vi "总磷氨氮测量流程.vi"(10 "量程模式":T1, 11 "参数":T2={"站号"=1, "量程切换"=enum."AUTO", "控制命令"=enum."启动测量", "模式设置"=enum."待机", "测量间隔"=0} {"站号" items=["总磷"=1, "总氮"=2]}) -> ()   [LabVIEW 2016, in "斯坦道仪器.lvlib"]
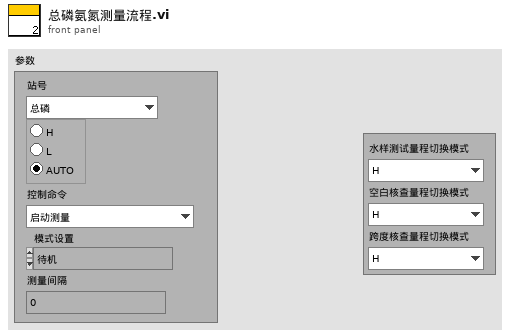
[diagram p1: front panel]
types:
  T1 = cluster{"水样测试量程切换模式":enum16{"H", "L", "AUTO"}, "空白核查量程切换模式":enum16{"H", "L", "AUTO"}, "跨度核查量程切换模式":enum16{"H", "L", "AUTO"}}
  T2 = cluster{"站号":u16, "量程切换":enum32{"H", "L", "AUTO"}, "控制命令":enum16{"启动测量", "标样核查", "零点核查", "跨度核查", "空白测试", "平行样测试", "加标回收", "空白校准", "标样校准", "初始化（清洗）", "停止测试", "仪器重启", "校时", "模式设置", "测量间隔设置"}, "模式设置":enum16{"待机", "连续模式", "周期模式", "定点模式", "受控模式", "手动模式"}, "测量间隔":u16}
  T3 = enum16{"初始化", "通电", "参数1启动", "等待参数1测试完成", "参数1测试完成", "参数1存储数据", "参数2启动", "等待参数2测试完成", "参数2测试完成", "参数2存储数据", "断电", "结束"}
  T4 = cluster{"时间标识":timestamp, "设备":string, "日志信息":string, "流程参数":string}
  T5 = cluster{"时间标识":timestamp, "监测值":sgl, "单位":u16, "数据标识":string, "因子编码":u32, "标样参考值":sgl, "F0":sgl, "F1":sgl, "F2":sgl, "F3":sgl, "F4":sgl, "F5":sgl, "F6":sgl, "F7":sgl, "X":sgl, "温度":sgl, "湿度":sgl, "量程标识":string}
  T6 = enum16{"维护数据", "水样测试", "标样核查", "零点核查", "跨度核查", "空白测试", "平行样测试", "加标回收", "空白校准", "标样校准", "初始化（清洗）"}
  T7 = cluster{"系统时间":timestamp, "工作状态":enum16{"空闲", "水样测试", "标样核查", "零点核查", "跨度核查", "空白测试", "平行样测试", "加标回收", "空白校准", "标样校准", "初始化（清洗）"}, "测量模式":enum16{"待机", "连续模式", "周期模式", "定点模式", "受控模式", "手动模式"}, "告警代码":enum16{"无告警", "缺试剂告警", "缺水样告警", "缺蒸馏水告警", "缺标液告警", "仪表漏液告警", "标定异常告警", "超量程告警", "加热异常", "低试剂预警", "超上限告警", "超下限告警", "仪表内部其他异常", "滴定异常告警", "电极异常告警", "量程切换告警", "参数设置告警", "PH电极电位异常", "电导率电极异常", "浊度光度异常", "溶解氧电极异常", "溶解氧光强异常", "温度异常告警", "PH异常告警", "溶解氧异常告警", "电导率异常告警", "浊度异常告警", "叶绿素异常告警", "藻密度异常告警", "蓝绿藻异常告警", "ORP异常告警", "氨氮异常告警", "清洁刷异常告警", "SD卡异常告警", "蓝牙异常告警", "Wifi异常告警", "流程异常告警"}, "故障代码":enum16{"无故障", "电机故障", "温度故障", "通讯故障", "滴定故障"}, "日志代码":u16, "软件版本":u16, "F0":sgl, "F1":sgl, "F2":sgl, "F3":sgl, "T":sgl, "H":sgl, "id":u16, "flowid":u16, "量程":u16, "总磷控温温度1":sgl, "营养盐控温温度2":sgl, "ADC":sgl}
  T8 = enum16{"启动测量", "标样核查", "零点核查", "跨度核查", "空白测试", "平行样测试", "加标回收", "空白校准", "标样校准", "初始化（清洗）", "停止测试", "仪器重启", "校时", "模式设置", "测量间隔设置"}
  T9 = enum16{"空闲", "水样测试", "标样核查", "零点核查", "跨度核查", "空白测试", "平行样测试", "加标回收", "空白校准", "标样校准", "初始化（清洗）"}
  T10 = cluster{"因子编码":u32, "单位":u16, "标样参考值":sgl, "水样数据时间":timestamp, "水样实测值":sgl, "水样数据标识":string, "标样数据时间":timestamp, "标样实测值":sgl, "标样数据标识":string, "空白数据时间":timestamp, "空白实测值":sgl, "空白数据标识":string, "零点核查数据时间":timestamp, "零点核查实测值":sgl, "零点核查数据标识":string, "跨度核查数据时间":timestamp, "跨度核查实测值":sgl, "跨度核查数据标识":string, "加标回收数据时间":timestamp, "加标回收实测值":sgl, "加标回收数据标识":string, "平行样数据时间":timestamp, "平行样实测值":sgl, "平行样数据标识":string, "F0":sgl, "F1":sgl, "F2":sgl, "F3":sgl, "F4":sgl, "F5":sgl, "F6":sgl, "F7":sgl, "温度":sgl, "湿度":sgl, "X值":sgl}
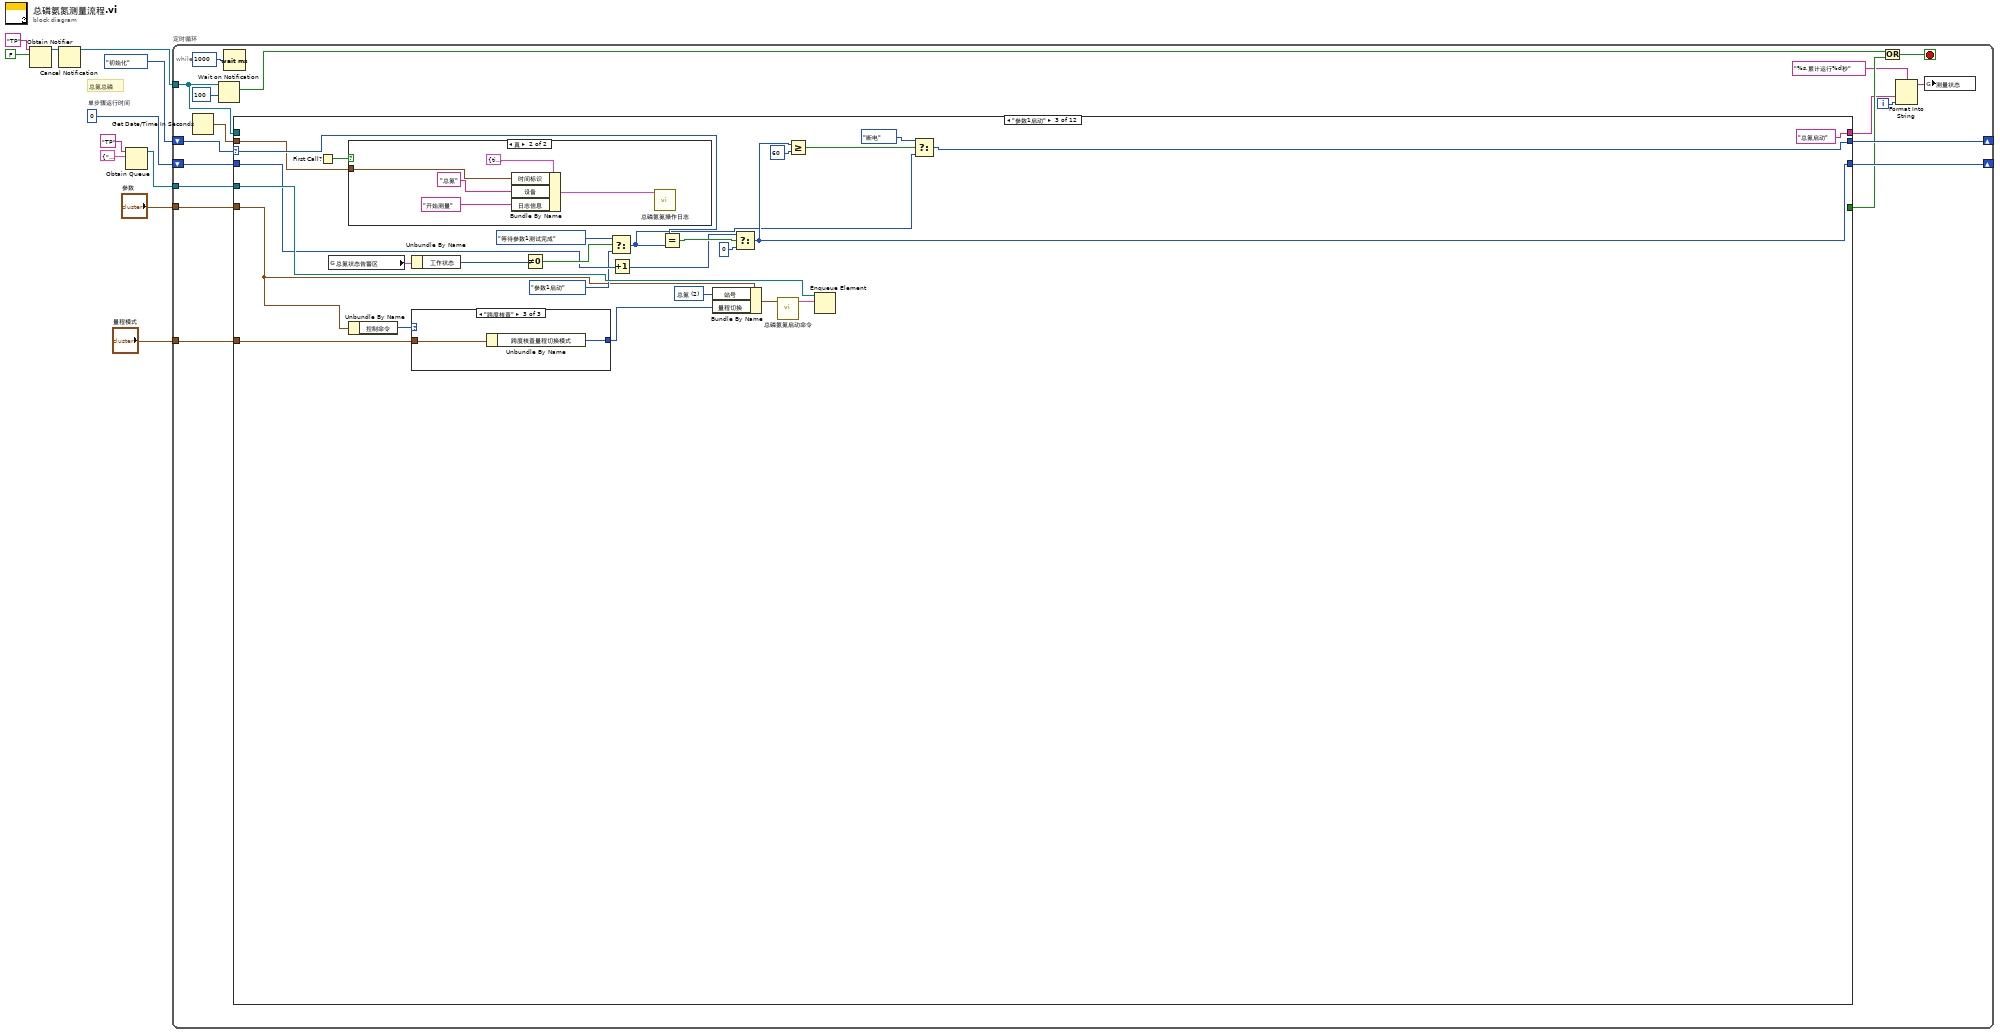
[diagram p0: block diagram]
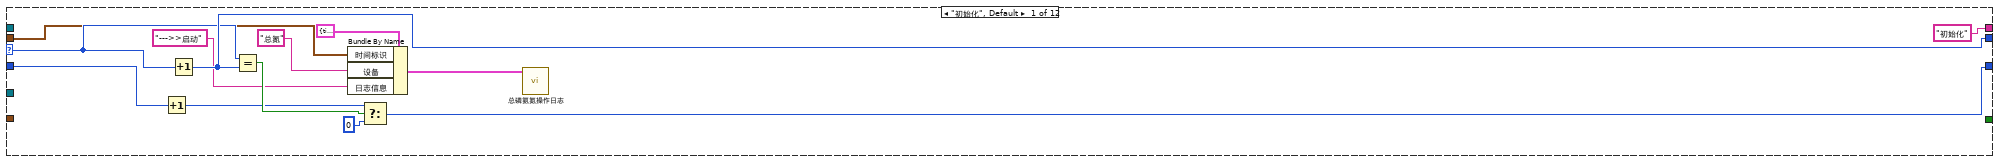
[diagram p2: hidden frame]
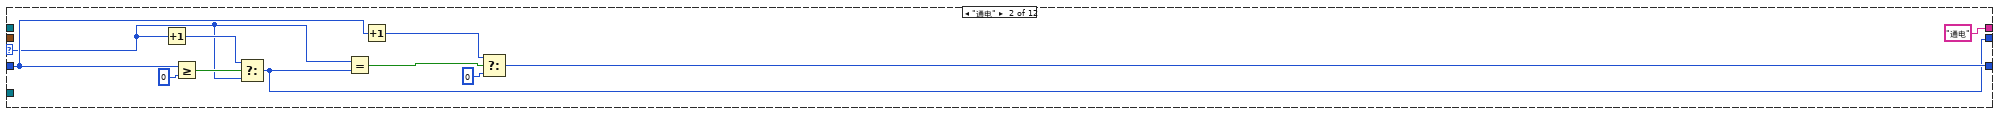
[diagram p3: hidden frame]
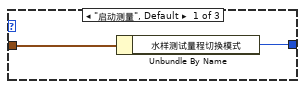
[diagram p4: hidden frame]
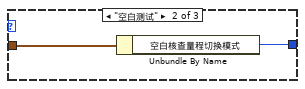
[diagram p5: hidden frame]
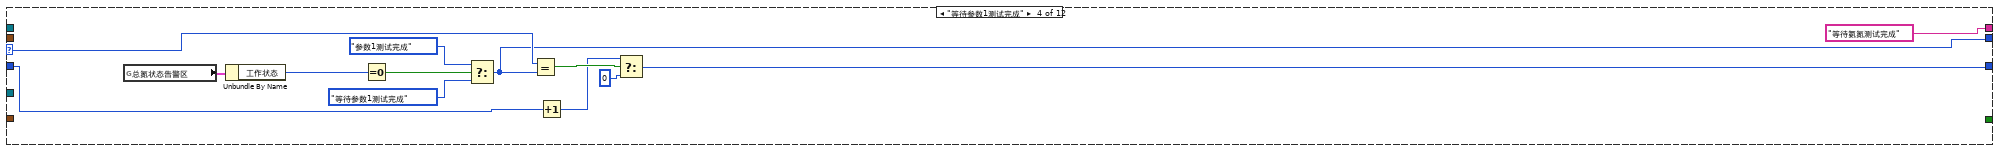
[diagram p7: hidden frame]
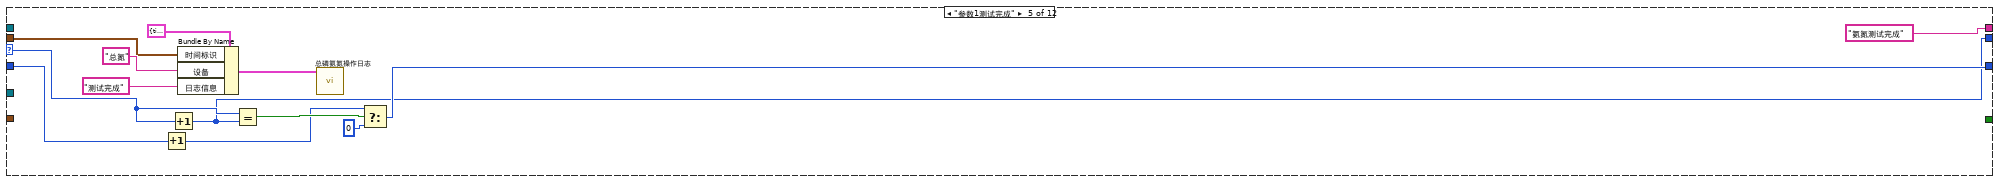
[diagram p8: hidden frame]
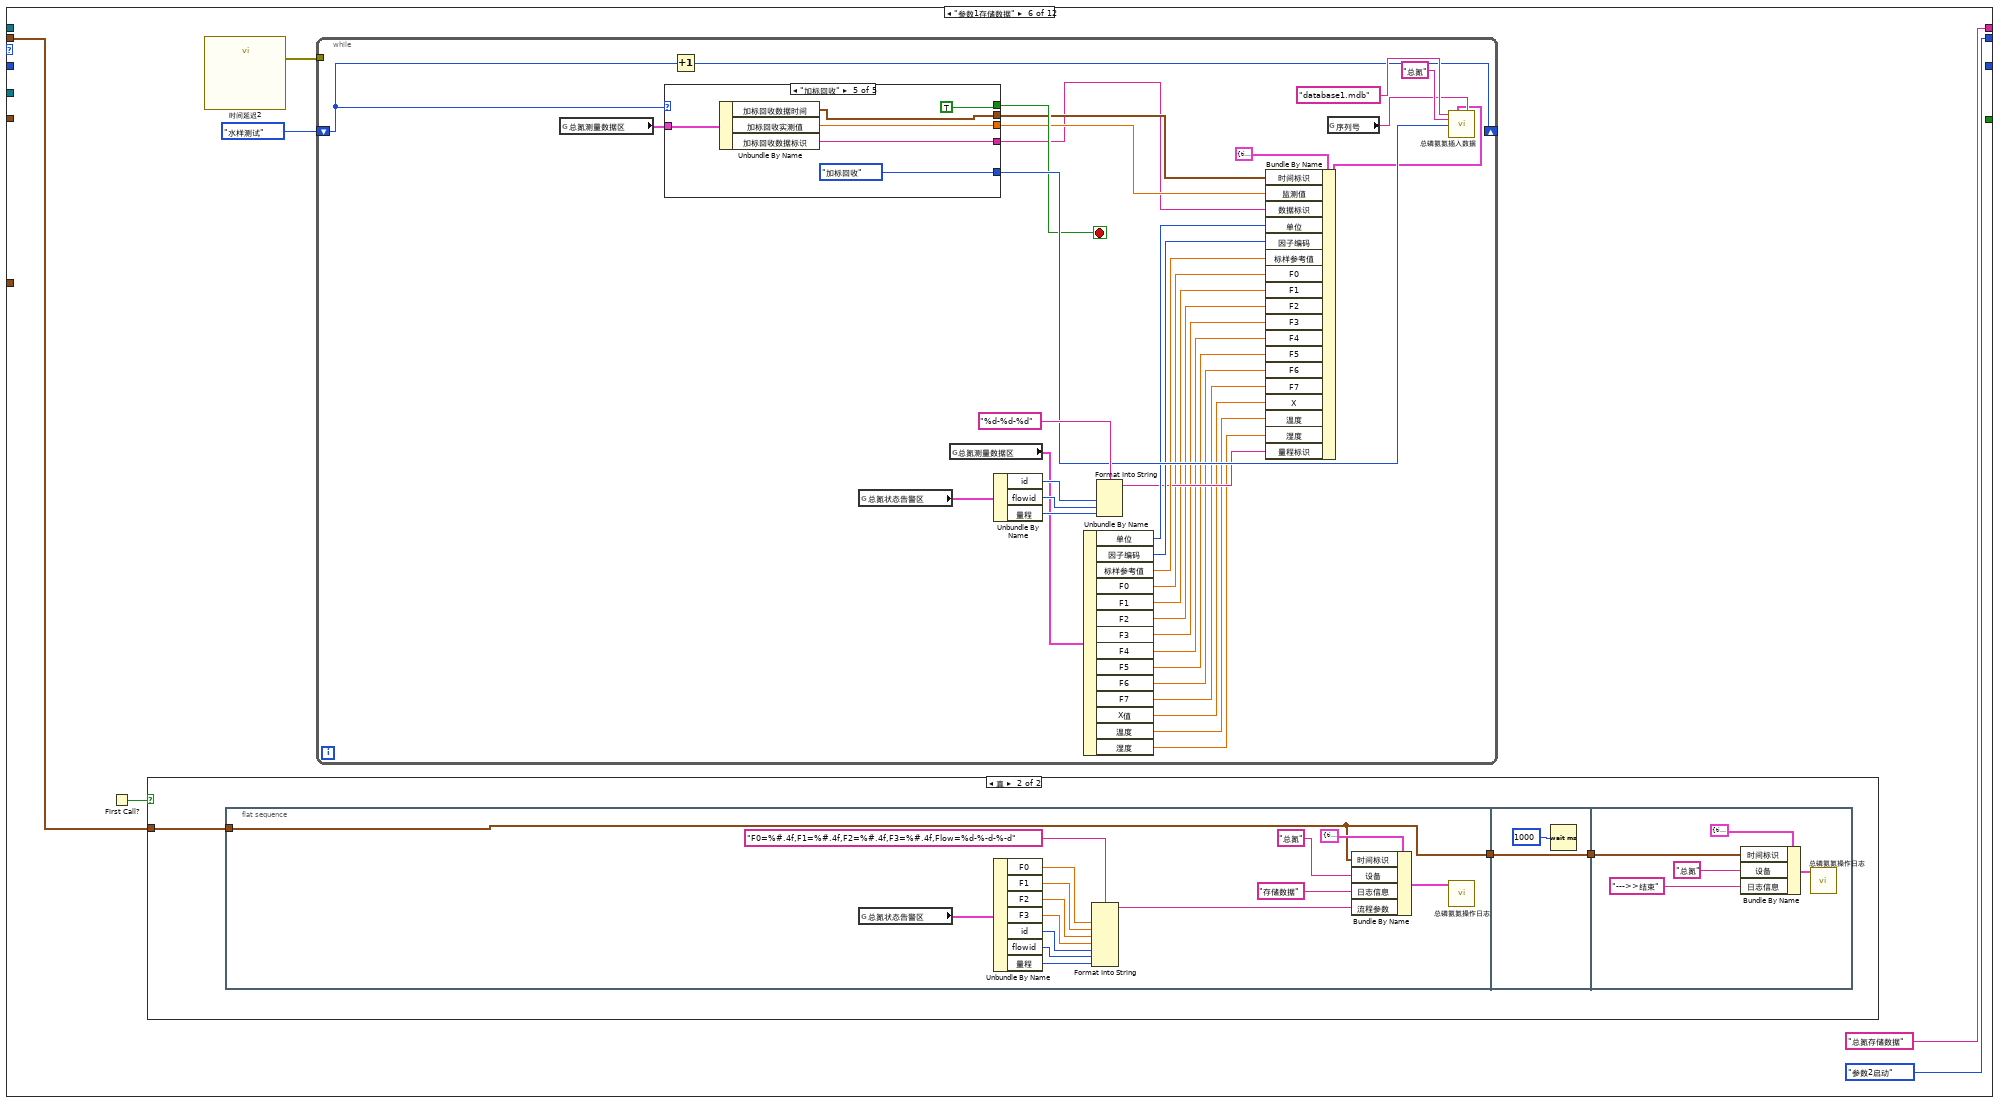
[diagram p9: hidden frame]
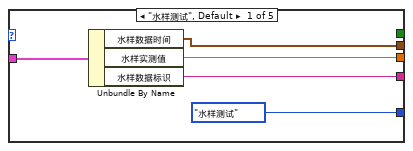
[diagram p10: hidden frame]
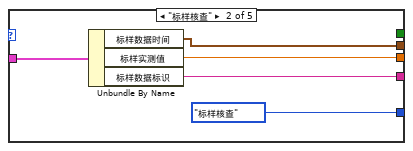
[diagram p11: hidden frame]
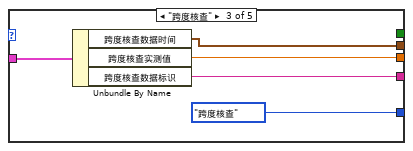
[diagram p12: hidden frame]
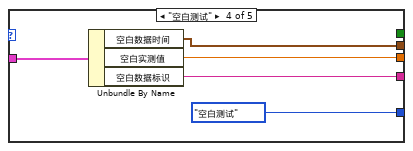
[diagram p13: hidden frame]
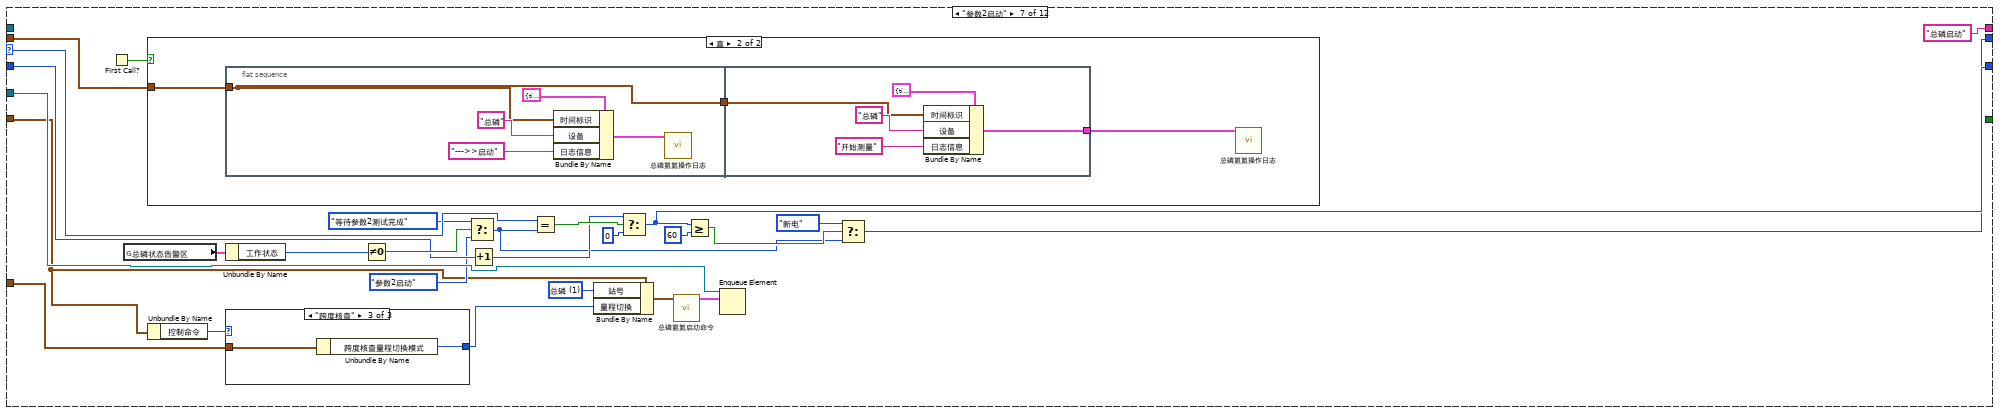
[diagram p15: hidden frame]
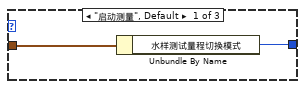
[diagram p16: hidden frame]
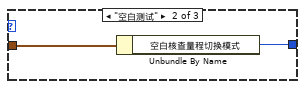
[diagram p17: hidden frame]
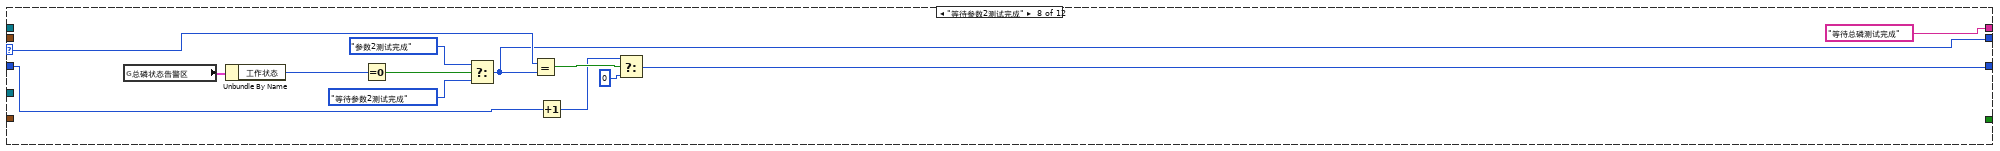
[diagram p19: hidden frame]
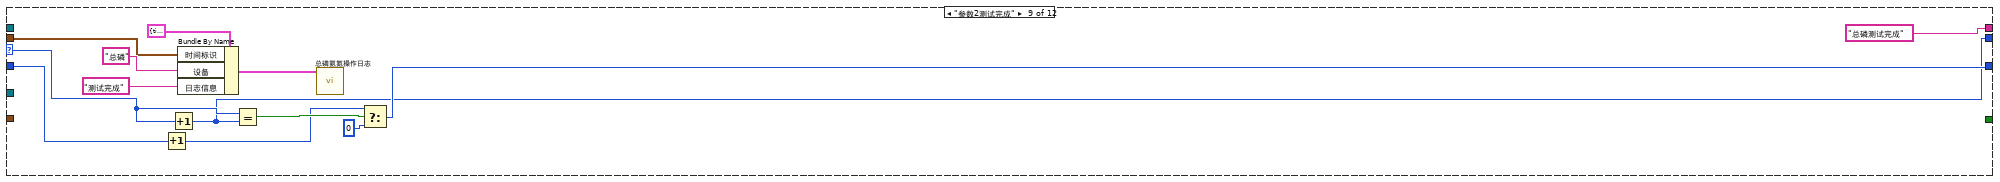
[diagram p20: hidden frame]
diagram:
  w7 = 0  # 单步骤运行时间
  # "总氮总磷"
  n1 = Obtain Notifier(name (unnamed)="TP" ("名称（未命名）"), notification data type=FALSE) -> (notifier out=w4:refnum<notifier>)  [unwired: 2 in, 2 out]
  n2 = Cancel Notification(0:w4) -> (8:w3:refnum<notifier>)  [unwired: 1 in, 2 out]
  n3 = Obtain Queue(name (unnamed)="TP" ("名称（未命名）"), element data type=cluster{"命令":string, "data":variant} {"命令"="", "data"=variant}) -> (queue out=w8:refnum<queue>)  [unwired: 3 in, 2 out]
  n4 = while "定时循环" {
    shift-right: [w28] -> _
    shift-left: T3."初始化" ("枚举") -> [w29]
    tunnel: w8 -> [w27]
    shift-right: [w25] -> _
    shift-left: w7 -> [w26]
    tunnel: w3 -> [w24]
    tunnel: "参数" -> [w19]
    tunnel: "量程模式" -> [w13]
    i -> [w15]
    stop <- w20 stop-if-true
    n5 = Get Date/Time In Seconds() -> (seconds since 1Jan1904=w17:timestamp)
    n6 = Wait on Notification(notifier=w24, timeout in ms (-1)=100 ("超时毫秒(-1)")) -> (notification=w21:bool)  [unwired: 2 in, 3 out]
    n7 = Wait (ms)(milliseconds to wait=u32 1000 ("等待时间（毫秒）")) -> ()  [unwired: 1 out]
    n8 = case shown="\"参数1启动\"" w29 {
      selector: w29 -> [w40 w47 w75 w99 w114 _ w224 w260 w276 _ w368 _]
      tunnel: [_ _ _ _ _ _ _ _ _ _ _ TRUE] -> w22
      tunnel: [w41 w46 w54 w98 w113 T3."参数2启动" ("枚举") w209 w258 w274 T3."断电" ("枚举") w367 T3."结束" ("枚举")] -> w28
      tunnel: w27 -> [_ _ w80 _ _ _ w232 _ _ _ _ w380]
      tunnel: w26 -> [w42 w48 w76 w101 w115 _ w225 w261 w277 _ w370 _]
      tunnel: [w38 w49 w59 w100 w116 _ w210 w259 w275 0 ("t") w369 0 ("t")] -> w25
      tunnel: w24 -> [_ _ _ _ _ _ _ _ _ _ _ w379]
      tunnel: w19 -> [_ _ w63 _ _ _ w218 _ _ _ _ _]
      tunnel: w17 -> [w31 _ w68 _ w106 w123 w223 _ w269 w286 _ w373]
      tunnel: ["初始化" ("输入 1") "通电" ("输入 1") "总氮启动" ("输入 1") "等待氨氮测试完成" ("输入 1") "氨氮测试完成" ("输入 1") "总氮存储数据" ("输入 1") "总磷启动" ("输入 1") "等待总磷测试完成" ("输入 1") "总磷测试完成" ("输入 1") "总磷存储数据" ("输入 1") "断电" ("输入 1") "结束" ("输入 1")] -> w14
      tunnel: w13 -> [_ _ w61 _ _ _ w216 _ _ _ _ _]
      frame "初始化", Default {
        n9 = Increment(x=w42) -> (x+1=w36:i32)
        n10 = Increment(x=w40) -> (x+1=w41:T3)
        n11 = Equal?(x=w40, y=w41) -> (x = y?=w39:bool)
        n12 = Bundle By Name(cluster=T4 {"时间标识"=timestamp(0 s since 1904-01-01), "设备"="", "日志信息"="", "流程参数"=""} ("data in"), "时间标识"=w31, "设备"="总氮", "日志信息"="--->>启动") -> (w35:T4)
        n13 = Select(t=w36, s=w39, f=0 ("t")) -> (s? t:f=w38:i32)
        n14 = call "总磷氨氮操作日志.vi"("data in"=w35) -> ()  [unwired: 11 in]
      }
      frame "通电" {
        n15 = Increment(x=w47) -> (x+1=w51:T3)
        n16 = Greater Or Equal?(x=w48, y=0) -> (x >= y?=w52:bool)
        n17 = Select(t=w51, s=w52, f=w47) -> (s? t:f=w46:T3)
        n18 = Equal?(x=w47, y=w46) -> (x = y?=w50:bool)
        n19 = Increment(x=w48) -> (x+1=w45:i32)
        n20 = Select(t=w45, s=w50, f=0 ("t")) -> (s? t:f=w49:i32)
      }
      frame "参数1启动" {
        w70 = u16 2 items=["总磷"=1, "总氮"=2, "氨氮"=3] ("站号")
        n21 = First Call?() -> (First Call?: T/F=w67:bool)
        n22 = global read "VAR总磷氨氮全局变量.vi" "总氮状态告警区"() -> (w69:T7)
        n23 = case shown="真" w67 {
          tunnel: w68 -> [_ w87]
          frame False {
          }
          frame True {
            n24 = Bundle By Name(cluster=T4 {"时间标识"=timestamp(0 s since 1904-01-01), "设备"="", "日志信息"="", "流程参数"=""} ("data in"), "时间标识"=w87, "设备"="总氮", "日志信息"="开始测量") -> (w91:T4)
            n25 = call "总磷氨氮操作日志.vi"("data in"=w91) -> ()  [unwired: 11 in]
          }
        }
        n26 = Unbundle By Name(w63) -> ("控制命令"=w62:T8)
        n27 = Unbundle By Name(w69) -> ("工作状态"=w79:T9)
        n28 = case shown="\"跨度核查\"" w62 {
          tunnel: w61 -> [w82 w84 w86]
          tunnel: [w81 w83 w85] -> w60
          frame "启动测量", Default {
            n29 = Unbundle By Name(w82) -> ("水样测试量程切换模式"=w81:enum16{"H", "L", "AUTO"})
          }
          frame "空白测试" {
            n30 = Unbundle By Name(w84) -> ("空白核查量程切换模式"=w83:enum16{"H", "L", "AUTO"})
          }
          frame "跨度核查" {
            n31 = Unbundle By Name(w86) -> ("跨度核查量程切换模式"=w85:enum16{"H", "L", "AUTO"})
          }
        }
        n32 = Not Equal To 0?(x=w79) -> (x != 0?=w78:bool)
        n33 = Select(t=T3."等待参数1测试完成" ("枚举"), s=w78, f=T3."参数1启动" ("枚举")) -> (s? t:f=w56:T3)
        n34 = Increment(x=w76) -> (x+1=w73:i32)
        n35 = Equal?(x=w75, y=w56) -> (x = y?=w77:bool)
        n36 = Bundle By Name(cluster=w63, "站号"=w70, "量程切换"=w60) -> (w71:T2)
        n37 = Select(t=w73, s=w77, f=0 ("t")) -> (s? t:f=w59:i32)
        n38 = call "总磷氨氮启动命令.vi"("参数"=w71) -> ("启动命令"=w72:cluster{"命令":string, "data":variant})  [unwired: 10 in]
        n39 = Greater Or Equal?(x=w59, y=60) -> (x >= y?=w57:bool)
        n40 = Enqueue Element(queue=w80, element=w72) -> ()  [unwired: 2 in, 3 out]
        n41 = Select(t=T3."断电" ("枚举"), s=w57, f=w56) -> (s? t:f=w54:T3)
      }
      frame "等待参数1测试完成" {
        n42 = global read "VAR总磷氨氮全局变量.vi" "总氮状态告警区"() -> (w95:T7)
        n43 = Unbundle By Name(w95) -> ("工作状态"=w104:T9)
        n44 = Equal To 0?(x=w104) -> (x = 0?=w103:bool)
        n45 = Select(t=T3."参数1测试完成" ("枚举"), s=w103, f=T3."等待参数1测试完成" ("枚举")) -> (s? t:f=w98:T3)
        n46 = Equal?(x=w99, y=w98) -> (x = y?=w102:bool)
        n47 = Increment(x=w101) -> (x+1=w96:i32)
        n48 = Select(t=w96, s=w102, f=0 ("t")) -> (s? t:f=w100:i32)
      }
      frame "参数1测试完成" {
        n49 = Increment(x=w115) -> (x+1=w111:i32)
        n50 = Increment(x=w114) -> (x+1=w113:T3)
        n51 = Bundle By Name(cluster=T4 {"时间标识"=timestamp(0 s since 1904-01-01), "设备"="", "日志信息"="", "流程参数"=""} ("data in"), "时间标识"=w106, "设备"="总氮", "日志信息"="测试完成") -> (w110:T4)
        n52 = Equal?(x=w114, y=w113) -> (x = y?=w117:bool)
        n53 = call "总磷氨氮操作日志.vi"("data in"=w110) -> ()  [unwired: 11 in]
        n54 = Select(t=w111, s=w117, f=0 ("t")) -> (s? t:f=w116:i32)
      }
      frame "参数1存储数据" {
        n55 = First Call?() -> (First Call?: T/F=w121:bool)
        n56 = case shown="真" w121 {
          tunnel: w123 -> [_ w186]
          frame False {
          }
          frame True {
            n57 = flat-sequence {
              tunnel: w186 -> [w197]
              tunnel: [w197] -> w185
              tunnel: w185 -> [w203]
              tunnel: [w203] -> w184
              tunnel: w184 -> [w204]
              frame #0 {
                n58 = global read "VAR总磷氨氮全局变量.vi" "总氮状态告警区"() -> (w196:T7)
                n59 = Unbundle By Name(w196) -> ("F0"=w188:sgl, "F1"=w189:sgl, "F2"=w190:sgl, "F3"=w191:sgl, "id"=w192:u16, "flowid"=w193:u16, "量程"=w194:u16)
                n60 = Format Into String(format string="F0=%#.4f,F1=%#.4f,F2=%#.4f,F3=%#.4f,Flow=%d-%-d-%-d" ("格式字符串"), w188, w189, w190, w191, w192, w193, w194) -> (resulting string=w187:string)  [unwired: 2 in, 1 out]
                n61 = Bundle By Name(cluster=T4 {"时间标识"=timestamp(0 s since 1904-01-01), "设备"="", "日志信息"="", "流程参数"=""} ("data in"), "时间标识"=w197, "设备"="总氮", "日志信息"="存储数据", "流程参数"=w187) -> (w201:T4)
                n62 = call "总磷氨氮操作日志.vi"("data in"=w201) -> ()  [unwired: 11 in]
              }
              frame #1 {
                n63 = Wait (ms)(milliseconds to wait=u32 1000 ("等待时间（毫秒）")) -> ()  [unwired: 1 out]
              }
              frame #2 {
                n64 = Bundle By Name(cluster=T4 {"时间标识"=timestamp(0 s since 1904-01-01), "设备"="", "日志信息"="", "流程参数"=""} ("data in"), "时间标识"=w204, "设备"="总氮", "日志信息"="--->>结束") -> (w205:T4)
                n65 = call "总磷氨氮操作日志.vi"("data in"=w205) -> ()  [unwired: 11 in]
              }
            }
          }
        }
        n66 = call "时间延迟2"() -> ("error out"=w118:errorcluster)  [unwired: 11 in]
        n67 = while {
          shift-right: [w145] -> _
          shift-left: enum16{"水样测试", "标样核查", "跨度核查", "空白测试", "加标回收"}."水样测试" ("测量模式") -> [w146]
          tunnel: w118 -> [_]
          stop <- w147 stop-if-true
          n68 = global read "VAR总磷氨氮全局变量.vi" "总氮测量数据区"() -> (w149:T10)
          n69 = case shown="\"加标回收\"" w146 {
            tunnel: w149 -> [w158 w163 w168 w173 w178]
            tunnel: [w162 w167 w172 w177 w183] -> w143
            tunnel: [w161 w166 w171 w176 w182] -> w142
            tunnel: [w160 w165 w170 w175 w181] -> w141
            tunnel: [T6."水样测试" ("测量模式") T6."标样核查" ("测量模式") T6."跨度核查" ("测量模式") T6."空白测试" ("测量模式") T6."加标回收" ("测量模式")] -> w148
            tunnel: [_ _ _ _ TRUE] -> w147
            frame "水样测试", Default {
              n70 = Unbundle By Name(w158) -> ("水样数据时间"=w162:timestamp, "水样实测值"=w161:sgl, "水样数据标识"=w160:string)
            }
            frame "标样核查" {
              n71 = Unbundle By Name(w163) -> ("标样数据时间"=w167:timestamp, "标样实测值"=w166:sgl, "标样数据标识"=w165:string)
            }
            frame "跨度核查" {
              n72 = Unbundle By Name(w168) -> ("跨度核查数据时间"=w172:timestamp, "跨度核查实测值"=w171:sgl, "跨度核查数据标识"=w170:string)
            }
            frame "空白测试" {
              n73 = Unbundle By Name(w173) -> ("空白数据时间"=w177:timestamp, "空白实测值"=w176:sgl, "空白数据标识"=w175:string)
            }
            frame "加标回收" {
              n74 = Unbundle By Name(w178) -> ("加标回收数据时间"=w183:timestamp, "加标回收实测值"=w182:sgl, "加标回收数据标识"=w181:string)
            }
          }
          n75 = Increment(x=w146) -> (x+1=w145:enum16{"水样测试", "标样核查", "跨度核查", "空白测试", "加标回收"})
          n76 = global read "VAR总磷氨氮全局变量.vi" "总氮状态告警区"() -> (w157:T7)
          n77 = global read "VAR总磷氨氮全局变量.vi" "总氮测量数据区"() -> (w144:T10)
          n78 = Unbundle By Name(w157) -> ("id"=w153:u16, "flowid"=w152:u16, "量程"=w151:u16)
          n79 = Unbundle By Name(w144) -> ("单位"=w140:u16, "因子编码"=w139:u32, "标样参考值"=w138:sgl, "F0"=w134:sgl, "F1"=w133:sgl, "F2"=w132:sgl, "F3"=w131:sgl, "F4"=w130:sgl, "F5"=w129:sgl, "F6"=w128:sgl, "F7"=w127:sgl, "X值"=w126:sgl, "温度"=w125:sgl, "湿度"=w124:sgl)
          n80 = Format Into String(format string="%d-%d-%d" ("格式字符串"), w153, w152, w151) -> (resulting string=w135:string)  [unwired: 2 in, 1 out]
          n81 = Bundle By Name(cluster=T5 {"时间标识"=timestamp(0 s since 1904-01-01), "监测值"=0.0, "单位"=0, "数据标识"="", "因子编码"=0, "标样参考值"=0.0, "F0"=0.0, "F1"=0.0, "F2"=0.0, "F3"=0.0, "F4"=0.0, "F5"=0.0, "F6"=0.0, "F7"=0.0, "X"=0.0, "温度"=0.0, "湿度"=0.0, "量程标识"=""} ("data"), "时间标识"=w143, "监测值"=w142, "数据标识"=w141, "单位"=w140, "因子编码"=w139, "标样参考值"=w138, "F0"=w134, "F1"=w133, "F2"=w132, "F3"=w131, "F4"=w130, "F5"=w129, "F6"=w128, "F7"=w127, "X"=w126, "温度"=w125, "湿度"=w124, "量程标识"=w135) -> (w136:T5)
          n82 = global read "VAR总磷氨氮全局变量.vi" "序列号"() -> (w150:string)
          n83 = call "总磷氨氮插入数据.vi"("database"="database1.mdb", "data"=w136, "SN"=w150, "table"="总氮", "测量模式"=w148) -> ()  [unwired: 10 in, 1 out]
        }
      }
      frame "参数2启动" {
        w233 = u16 1 items=["总氮"=2, "总磷"=1] ("站号")
        n84 = First Call?() -> (First Call?: T/F=w222:bool)
        n85 = global read "VAR总磷氨氮全局变量.vi" "总磷状态告警区"() -> (w226:T7)
        n86 = case shown="真" w222 {
          tunnel: w223 -> [_ w242]
          frame False {
          }
          frame True {
            n87 = flat-sequence {
              tunnel: w242 -> [w245]
              tunnel: [w245] -> w243
              tunnel: [w254] -> w244
              tunnel: w243 -> [w250]
              frame #0 {
                n88 = Bundle By Name(cluster=T4 {"时间标识"=timestamp(0 s since 1904-01-01), "设备"="", "日志信息"="", "流程参数"=""} ("data in"), "时间标识"=w245, "设备"="总磷", "日志信息"="--->>启动") -> (w249:T4)
                n89 = call "总磷氨氮操作日志.vi"("data in"=w249) -> ()  [unwired: 11 in]
              }
              frame #1 {
                n90 = Bundle By Name(cluster=T4 {"时间标识"=timestamp(0 s since 1904-01-01), "设备"="", "日志信息"="", "流程参数"=""} ("data in"), "时间标识"=w250, "设备"="总磷", "日志信息"="开始测量") -> (w254:T4)
              }
            }
            n91 = call "总磷氨氮操作日志.vi"("data in"=w244) -> ()  [unwired: 11 in]
          }
        }
        n92 = Unbundle By Name(w218) -> ("控制命令"=w217:T8)
        n93 = Unbundle By Name(w226) -> ("工作状态"=w231:T9)
        n94 = case shown="\"跨度核查\"" w217 {
          tunnel: w216 -> [w237 w239 w241]
          tunnel: [w236 w238 w240] -> w215
          frame "启动测量", Default {
            n95 = Unbundle By Name(w237) -> ("水样测试量程切换模式"=w236:enum16{"H", "L", "AUTO"})
          }
          frame "空白测试" {
            n96 = Unbundle By Name(w239) -> ("空白核查量程切换模式"=w238:enum16{"H", "L", "AUTO"})
          }
          frame "跨度核查" {
            n97 = Unbundle By Name(w241) -> ("跨度核查量程切换模式"=w240:enum16{"H", "L", "AUTO"})
          }
        }
        n98 = Not Equal To 0?(x=w231) -> (x != 0?=w230:bool)
        n99 = Select(t=T3."等待参数2测试完成" ("枚举"), s=w230, f=T3."参数2启动" ("枚举")) -> (s? t:f=w211:T3)
        n100 = Increment(x=w225) -> (x+1=w227:i32)
        n101 = Equal?(x=w224, y=w211) -> (x = y?=w229:bool)
        n102 = Bundle By Name(cluster=w218, "站号"=w233, "量程切换"=w215) -> (w234:T2)
        n103 = Select(t=w227, s=w229, f=0 ("t")) -> (s? t:f=w210:i32)
        n104 = call "总磷氨氮启动命令.vi"("参数"=w234) -> ("启动命令"=w235:cluster{"命令":string, "data":variant})  [unwired: 10 in]
        n105 = Greater Or Equal?(x=w210, y=60) -> (x >= y?=w213:bool)
        n106 = Enqueue Element(queue=w232, element=w235) -> ()  [unwired: 2 in, 3 out]
        n107 = Select(t=T3."断电" ("枚举"), s=w213, f=w211) -> (s? t:f=w209:T3)
      }
      frame "等待参数2测试完成" {
        n108 = global read "VAR总磷氨氮全局变量.vi" "总磷状态告警区"() -> (w262:T7)
        n109 = Unbundle By Name(w262) -> ("工作状态"=w267:T9)
        n110 = Equal To 0?(x=w267) -> (x = 0?=w266:bool)
        n111 = Select(t=T3."参数2测试完成" ("枚举"), s=w266, f=T3."等待参数2测试完成" ("枚举")) -> (s? t:f=w258:T3)
        n112 = Equal?(x=w260, y=w258) -> (x = y?=w265:bool)
        n113 = Increment(x=w261) -> (x+1=w263:i32)
        n114 = Select(t=w263, s=w265, f=0 ("t")) -> (s? t:f=w259:i32)
      }
      frame "参数2测试完成" {
        n115 = Increment(x=w277) -> (x+1=w278:i32)
        n116 = Increment(x=w276) -> (x+1=w274:T3)
        n117 = Bundle By Name(cluster=T4 {"时间标识"=timestamp(0 s since 1904-01-01), "设备"="", "日志信息"="", "流程参数"=""} ("data in"), "时间标识"=w269, "设备"="总磷", "日志信息"="测试完成") -> (w273:T4)
        n118 = Equal?(x=w276, y=w274) -> (x = y?=w280:bool)
        n119 = call "总磷氨氮操作日志.vi"("data in"=w273) -> ()  [unwired: 11 in]
        n120 = Select(t=w278, s=w280, f=0 ("t")) -> (s? t:f=w275:i32)
      }
      frame "参数2存储数据" {
        n121 = First Call?() -> (First Call?: T/F=w283:bool)
        n122 = case shown="真" w283 {
          tunnel: w286 -> [_ w358]
          frame False {
          }
          frame True {
            n123 = global read "VAR总磷氨氮全局变量.vi" "总磷状态告警区"() -> (w357:T7)
            n124 = Unbundle By Name(w357) -> ("F0"=w349:sgl, "F1"=w350:sgl, "F2"=w351:sgl, "F3"=w352:sgl, "id"=w353:u16, "flowid"=w354:u16, "量程"=w355:u16)
            n125 = Format Into String(format string="F0=%#.4f,F1=%#.4f,F2=%#.4f,F3=%#.4f,Flow=%d-%-d-%-d" ("格式字符串"), w349, w350, w351, w352, w353, w354, w355) -> (resulting string=w348:string)  [unwired: 2 in, 1 out]
            n126 = Bundle By Name(cluster=T4 {"时间标识"=timestamp(0 s since 1904-01-01), "设备"="", "日志信息"="", "流程参数"=""} ("data in"), "时间标识"=w358, "设备"="总磷", "日志信息"="存储数据", "流程参数"=w348) -> (w362:T4)
            n127 = call "总磷氨氮操作日志.vi"("data in"=w362) -> ()  [unwired: 11 in]
          }
        }
        n128 = call "时间延迟"() -> ("error out"=w281:errorcluster)  [unwired: 11 in]
        n129 = while {
          shift-right: [w304] -> _
          shift-left: enum16{"水样测试", "标样核查", "跨度核查", "空白测试", "加标回收"}."水样测试" ("测量模式") -> [w305]
          tunnel: w281 -> [_]
          stop <- w306 stop-if-true
          n130 = global read "VAR总磷氨氮全局变量.vi" "总磷测量数据区"() -> (w303:T10)
          n131 = case shown="\"空白测试\"" w305 {
            tunnel: w303 -> [w326 w331 w336 w341 w347]
            tunnel: [w325 w330 w335 w340 w346] -> w310
            tunnel: [w324 w329 w334 w339 w345] -> w309
            tunnel: [w323 w328 w333 w338 w344] -> w308
            tunnel: [T6."水样测试" ("测量模式") T6."标样核查" ("测量模式") T6."跨度核查" ("测量模式") T6."空白测试" ("测量模式") T6."加标回收" ("测量模式")] -> w307
            tunnel: [_ _ _ _ TRUE] -> w306
            frame "水样测试", Default {
              n132 = Unbundle By Name(w326) -> ("水样数据时间"=w325:timestamp, "水样实测值"=w324:sgl, "水样数据标识"=w323:string)
            }
            frame "标样核查" {
              n133 = Unbundle By Name(w331) -> ("标样数据时间"=w330:timestamp, "标样实测值"=w329:sgl, "标样数据标识"=w328:string)
            }
            frame "跨度核查" {
              n134 = Unbundle By Name(w336) -> ("跨度核查数据时间"=w335:timestamp, "跨度核查实测值"=w334:sgl, "跨度核查数据标识"=w333:string)
            }
            frame "空白测试" {
              n135 = Unbundle By Name(w341) -> ("空白数据时间"=w340:timestamp, "空白实测值"=w339:sgl, "空白数据标识"=w338:string)
            }
            frame "加标回收" {
              n136 = Unbundle By Name(w347) -> ("加标回收数据时间"=w346:timestamp, "加标回收实测值"=w345:sgl, "加标回收数据标识"=w344:string)
            }
          }
          n137 = Increment(x=w305) -> (x+1=w304:enum16{"水样测试", "标样核查", "跨度核查", "空白测试", "加标回收"})
          n138 = global read "VAR总磷氨氮全局变量.vi" "总磷状态告警区"() -> (w318:T7)
          n139 = global read "VAR总磷氨氮全局变量.vi" "总磷测量数据区"() -> (w302:T10)
          n140 = Unbundle By Name(w318) -> ("id"=w314:u16, "flowid"=w313:u16, "量程"=w312:u16)
          n141 = Unbundle By Name(w302) -> ("单位"=w321:u16, "因子编码"=w320:u32, "标样参考值"=w319:sgl, "F0"=w288:sgl, "F1"=w289:sgl, "F2"=w290:sgl, "F3"=w291:sgl, "F4"=w292:sgl, "F5"=w293:sgl, "F6"=w294:sgl, "F7"=w295:sgl, "X值"=w296:sgl, "温度"=w297:sgl, "湿度"=w298:sgl)
          n142 = Format Into String(format string="%d-%d-%d" ("格式字符串"), w314, w313, w312) -> (resulting string=w299:string)  [unwired: 2 in, 1 out]
          n143 = Bundle By Name(cluster=T5 {"时间标识"=timestamp(0 s since 1904-01-01), "监测值"=0.0, "单位"=0, "数据标识"="", "因子编码"=0, "标样参考值"=0.0, "F0"=0.0, "F1"=0.0, "F2"=0.0, "F3"=0.0, "F4"=0.0, "F5"=0.0, "F6"=0.0, "F7"=0.0, "X"=0.0, "温度"=0.0, "湿度"=0.0, "量程标识"=""} ("data"), "时间标识"=w310, "监测值"=w309, "数据标识"=w308, "单位"=w321, "因子编码"=w320, "标样参考值"=w319, "F0"=w288, "F1"=w289, "F2"=w290, "F3"=w291, "F4"=w292, "F5"=w293, "F6"=w294, "F7"=w295, "X"=w296, "温度"=w297, "湿度"=w298, "量程标识"=w299) -> (w301:T5)
          n144 = global read "VAR总磷氨氮全局变量.vi" "序列号"() -> (w311:string)
          n145 = call "总磷氨氮插入数据.vi"("database"="database1.mdb", "data"=w301, "SN"=w311, "table"="总磷", "测量模式"=w307) -> ()  [unwired: 10 in, 1 out]
        }
      }
      frame "断电" {
        n146 = Increment(x=w370) -> (x+1=w363:i32)
        n147 = Increment(x=w368) -> (x+1=w367:T3)
        n148 = Equal?(x=w368, y=w367) -> (x = y?=w365:bool)
        n149 = Select(t=w363, s=w365, f=0 ("t")) -> (s? t:f=w369:i32)
      }
      frame "结束" {
        n150 = Release Queue(queue=w380) -> ()  [unwired: 2 in, 3 out]
        n151 = Cancel Notification(0:w379) -> (8:w378:refnum<notifier>)  [unwired: 1 in, 2 out]
        n152 = Release Notifier(notifier=w378) -> ()  [unwired: 2 in, 3 out]
        n153 = Bundle By Name(cluster=T4 {"时间标识"=timestamp(0 s since 1904-01-01), "设备"="", "日志信息"="", "流程参数"=""} ("data in"), "时间标识"=w373, "设备"="总磷", "日志信息"="--->>结束") -> (w377:T4)
        n154 = call "总磷氨氮操作日志.vi"("data in"=w377) -> ()  [unwired: 11 in]
      }
    }
    n155 = Or(x=w21, y=w22) -> (x .or. y?=w20:bool)
    n156 = Format Into String(format string="%s,累计运行%d秒" ("格式字符串"), w14, w15) -> (resulting string=w12:string)  [unwired: 2 in, 1 out]
    n157 = global write "VAR总磷氨氮全局变量.vi" "测量状态"(w12) -> ()
  }
